vi "tm_getcamerainfo.vi"(8 "error in (no error)":errorcluster, 10 "Info ID":u32(ring)=67109121 items=["BUS"=67109121, "CAMERA ID"=67109122, "VENDOR"=67109123, "MODEL"=67109124, "CAMERA VERSION"=67109125, "DRIVER VERSION"=67109126, "MODULE VERSIOIN"=67109127, "DCAMAPI VERSION"=67109128], 11 "Handle in":u32) -> (0 "error out":errorcluster, 2 "String":string, 3 "Handle out":u32)   [LabVIEW 2015]
uses:
  tmcamcon.dll
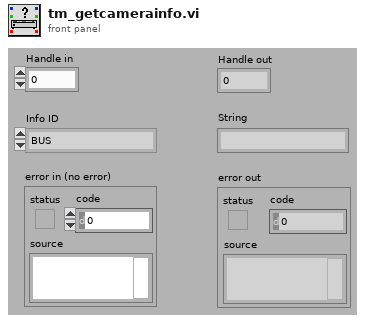
[diagram p1: front panel]
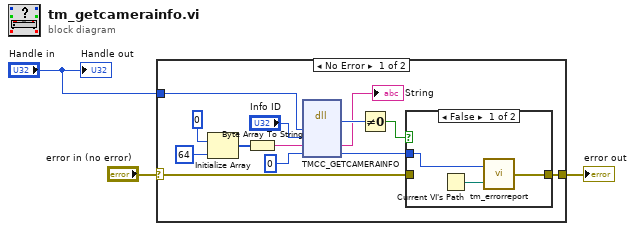
[diagram p0: block diagram]
diagram:
  n1 = case shown="No Error" "error in (no error)" {
    selector: "error in (no error)" -> [w7 w21]
    tunnel: [w4 w21] -> w2
    tunnel: "Handle in" -> [w8 _]
    frame No Error {
      n2 = Initialize Array(u8 0, 64) -> (w15:u8[])
      n3 = Byte Array To String(unsigned byte array=w15) -> (string=w12:string)
      n4 = dll-call lib="tmcamcon.dll" fn="TMCC_GETCAMERAINFO"("index"=w8, "ID"="Info ID", "string"=w12, "Erval"=0) -> ("return type"=w16:u32, "string"=→"String":string, "Erval"=w6:i32)  [unwired: 5 in, 2 out]
      n5 = Not Equal To 0?(x=w16) -> (x != 0?=w5:bool)
      n6 = case shown="False" w5 {
        tunnel: w7 -> [_ w20]
        tunnel: [w18 w20] -> w4
        tunnel: w6 -> [w17 _]
        frame False {
          n7 = Current VI's Path() -> (path=w19:path)
          n8 = call "tm_errorreport.vi"("Source"=w19, "Error"=w17) -> ("error out"=w18:errorcluster)
        }
        frame True {
        }
      }
    }
    frame Error {
    }
  }
  "error out" <- w2
  "Handle out" <- "Handle in"
